vi "Network_Check.vi"   [LabVIEW 2010]
uses:
  Anemometry/Anemometry Sub Vis/Globals/Constants_global.vi
  ADAM_Global.vi
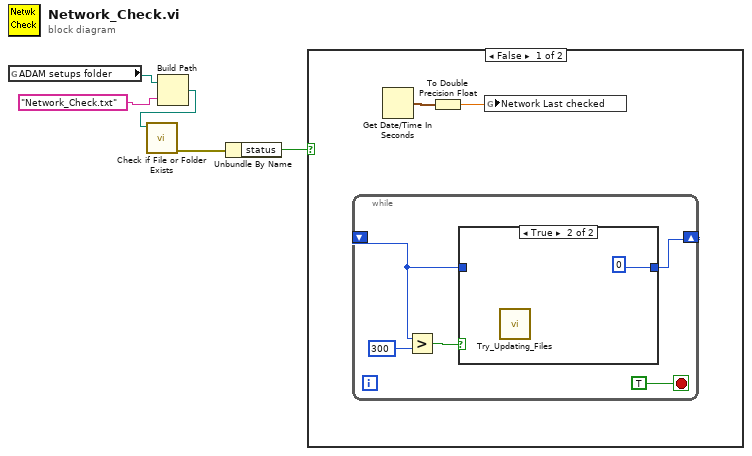
[diagram p0: block diagram]
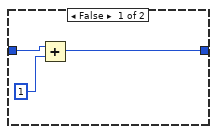
[diagram p2: hidden frame]
diagram:
  n1 = global read "Constants_global.vi" "ADAM setups folder"() -> (w3:path)
  n2 = Build Path(base path=w3, name or relative path="Network_Check.txt") -> (appended path=w2:path)
  n3 = call <vilib>:"Check if File or Folder Exists.vi"("path"=w2) -> ("error out"=w5:errorcluster)  [unwired: 2 in, 8 out]
  n4 = Unbundle By Name(w5) -> ("status"=w1:bool)
  n5 = case shown="False" w1 {
    frame False {
      n6 = while {
        shift-right: [w12] -> _
        shift-left: _ -> [w11]
        stop <- TRUE stop-if-true
        n7 = Greater?(x=w11, y=300) -> (0:w9:bool)
        n8 = case shown="True" w9 {
          tunnel: w11 -> [w15 _]
          tunnel: [w14 0] -> w12
          frame False {
            n9 = Add(x=w15, y=1) -> (x+y=w14:i32)
          }
          frame True {
            n10 = call "Try_Updating_Files.vi"() -> ()  [unwired: 4 out]
          }
        }
      }
      n11 = Get Date/Time In Seconds() -> (seconds since 1Jan1904=w7:timestamp)
      n12 = To Double Precision Float(number=w7) -> (double precision float=w6:dbl)
      n13 = global write "ADAM_Global.vi" "Network Last checked"(w6) -> ()
    }
    frame True {
    }
  }
